vi "Dpc Put Tms Tdi Bits.vi"(0 "hif":u32, 1 "cbit":i32, 2 "rgbSnd":string, 3 "fReturnTdo":i32, 4 "rgbRcv":string, 5 "perc":i32, 6 "ptrid":u16, 7 "error in (no error)":errorcluster) -> (20 "hif out":u32, 21 "function return":i32, 22 "rgbSnd out":string, 24 "rgbRcv out":string, 25 "perc out":i32, 26 "ptrid out":u16, 27 "error out":errorcluster)   [LabVIEW 2011, in "LVH-Adept.lvlib" / "DPCUTIL.lvlib"]
doc: "DPCAPI BOOL DpcPutTmsTdiBits(HANDLE hif, INT32 cbit, BYTE * rgbSnd, BOOL fReturnTdo, BYTE * rgbRcv, ERC * perc, TRID * ptrid);"
uses:
  DPCUTIL.lvlib
  Resources/dpcutil.dll
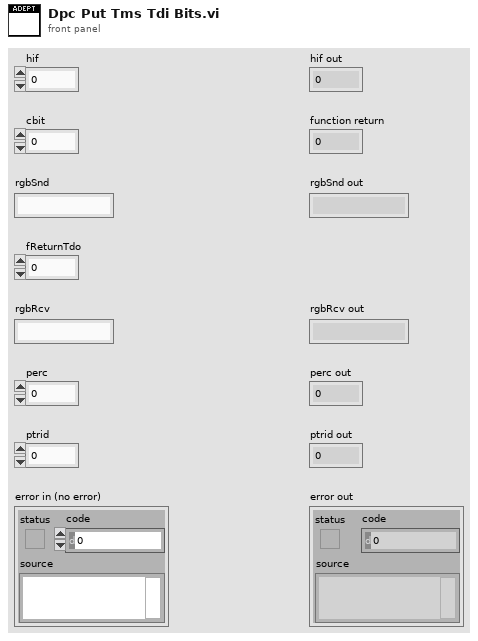
[diagram p1: front panel]
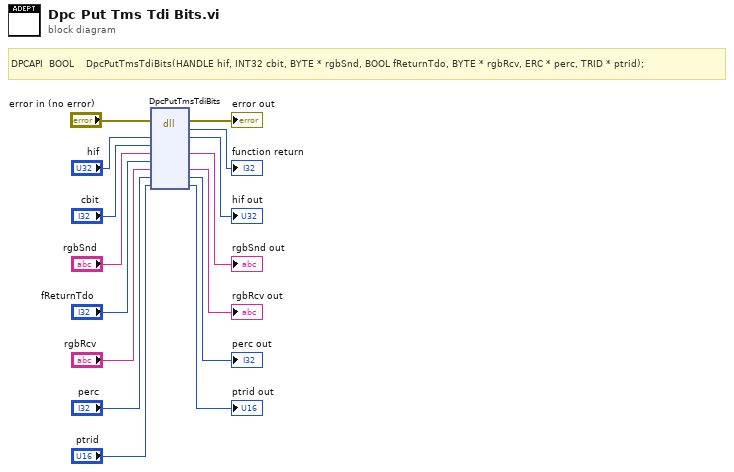
[diagram p0: block diagram]
diagram:
  # "DPCAPI  BOOL    DpcPutTmsTdiBits(HANDLE hif, INT32 cbit, BYTE * rgbSnd, BOOL fReturnTdo, BYTE * rgbRcv, ERC * perc, TRID * ptrid);"
  n1 = dll-call lib="C:/github/labviewhacker/LVH-Adept/LabVIEW/vi.lib/LabVIEW Hacker/Adept/Private/Resources/dpcutil.*" fn="DpcPutTmsTdiBits"(error in="error in (no error)", "hif"="hif", "cbit"="cbit", "rgbSnd"="rgbSnd", "fReturnTdo"="fReturnTdo", "rgbRcv"="rgbRcv", "perc"="perc", "ptrid"="ptrid") -> (error out=→"error out":errorcluster, →"function return":i32, "hif"=→"hif out":u32, "rgbSnd"=→"rgbSnd out":string, "rgbRcv"=→"rgbRcv out":string, "perc"=→"perc out":i32, "ptrid"=→"ptrid out":u16)  [unwired: 4 in, 1 out]
